vi "BrakeDelay (3).vi"(11 "Mtr Power":dbl) -> ()   [LabVIEW 2016]
uses:
  <vilib>/Rock Robotics/WPI/ThirdParty/CanMotor/TalonSRX/WPI_CANTalonSRX_BrakeOverride.ctl
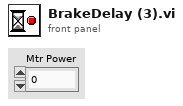
[diagram p1: front panel]
types:
  T1 = typedef "WPI_MotorControlDeviceRef.ctl" = cluster{"DeviceStatus":errorcluster, "Type":T2, "PWM":cluster{"PWM Channel":T3, "DeadBand":T4}, "CAN":cluster{"Device Number":u8, "SetOutput VI Ref":variant, "GetOutput VI Ref":variant, "Enable VI Ref":variant, "Disable VI Ref":variant, "Data":variant}, "Invert":bool}
  T2 = typedef "WPI_MotorControlType.ctl" = enum16{"PWM", "CAN"}
  T3 = typedef "FPGA_DIOPWMChannel.ctl" = enum8{"PWM 0", "PWM 1", "PWM 2", "PWM 3", "PWM 4", "PWM 5", "PWM 6", "PWM 7", "PWM 8", "PWM 9", "PWM MXP 0", "PWM MXP 1", "PWM MXP 2", "PWM MXP 3", "PWM MXP 4", "PWM MXP 5", "PWM MXP 6", "PWM MXP 7", "PWM MXP 8", "PWM MXP 9", "Invalid"}
  T4 = typedef "WPI_PWMDeadband.ctl" = cluster{"Name":string, "maxPositivePwm":i32, "minPositivePwm":i32, "centerPwm":i32, "maxNegativePwm":i32, "minNegativePwm":i32, "angularRange":u16}
  T5 = typedef "WPI_CANTalonSRX_BrakeOverride.ctl" = enum8{"No Override", "Override to Coast", "Override to Brake"}
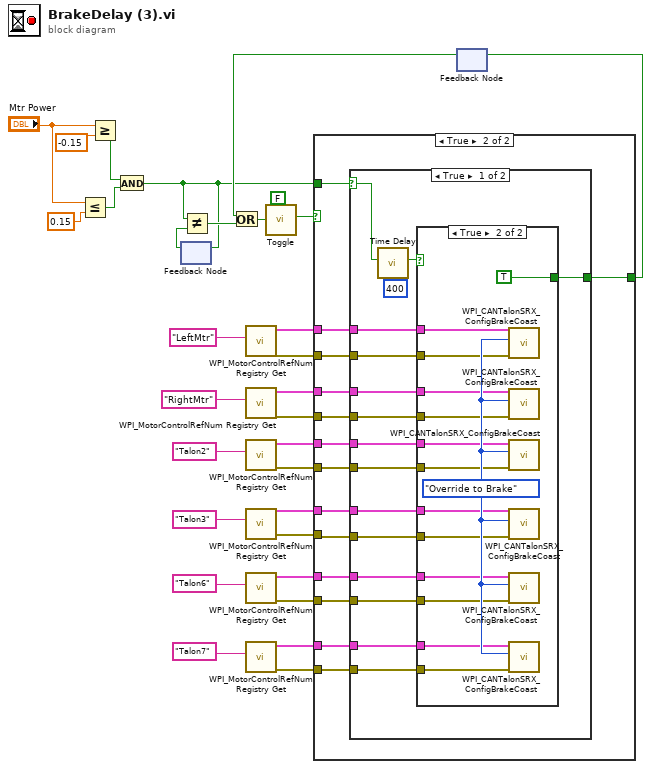
[diagram p0: block diagram]
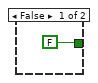
[diagram p2: hidden frame]
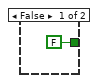
[diagram p3: hidden frame]
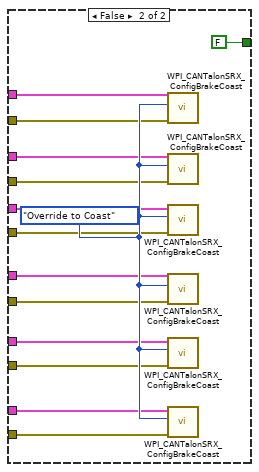
[diagram p4: hidden frame]
diagram:
  n1 = Less Or Equal?(x="Mtr Power", y=0.15) -> (x <= y?=w10:bool)
  n2 = Greater Or Equal?(x="Mtr Power", y=-0.15) -> (x >= y?=w9:bool)
  n3 = And(x=w9, y=w10) -> (x .and. y?=w2:bool)
  n4 = feedback #1() -> (w8:bool)  [unwired: 1 in]
  n5 = feedback-in #1(w2) -> ()
  n6 = Not Equal?(x=w2, y=w8) -> (x != y?=w7:bool)
  n7 = call <vilib>:"WPI_MotorControlRefNum Registry Get.vi"("refnum name"="LeftMtr") -> ("error out"=w30:errorcluster, "MotorControlDevRef"=w31:T1)  [unwired: 9 in]
  n8 = call <vilib>:"WPI_MotorControlRefNum Registry Get.vi"("refnum name"="RightMtr") -> ("error out"=w28:errorcluster, "MotorControlDevRef"=w29:T1)  [unwired: 9 in]
  n9 = call <vilib>:"WPI_MotorControlRefNum Registry Get.vi"("refnum name"="Talon2") -> ("error out"=w26:errorcluster, "MotorControlDevRef"=w27:T1)  [unwired: 9 in]
  n10 = call <vilib>:"WPI_MotorControlRefNum Registry Get.vi"("refnum name"="Talon3") -> ("error out"=w21:errorcluster, "MotorControlDevRef"=w20:T1)  [unwired: 9 in]
  n11 = call <vilib>:"WPI_MotorControlRefNum Registry Get.vi"("refnum name"="Talon6") -> ("error out"=w24:errorcluster, "MotorControlDevRef"=w25:T1)  [unwired: 9 in]
  n12 = call <vilib>:"WPI_MotorControlRefNum Registry Get.vi"("refnum name"="Talon7") -> ("error out"=w22:errorcluster, "MotorControlDevRef"=w23:T1)  [unwired: 9 in]
  n13 = feedback #2() -> (w3:bool)  [unwired: 1 in]
  n14 = Or(x=w3, y=w7) -> (x .or. y?=w6:bool)
  n15 = call "Toggle.vi"("Control"=FALSE, "Input"=w6) -> ("Output"=w5:bool)  [unwired: 9 in]
  n16 = case shown="True" w5 {
    tunnel: w20 -> [_ w41]
    tunnel: w21 -> [_ w42]
    tunnel: w22 -> [_ w46]
    tunnel: w23 -> [_ w45]
    tunnel: w24 -> [_ w44]
    tunnel: w25 -> [_ w43]
    tunnel: w26 -> [_ w40]
    tunnel: w27 -> [_ w39]
    tunnel: w28 -> [_ w38]
    tunnel: w29 -> [_ w37]
    tunnel: w30 -> [_ w36]
    tunnel: w31 -> [_ w35]
    tunnel: [FALSE w34] -> w4
    tunnel: w2 -> [_ w33]
    frame False {
    }
    frame True {
      n17 = case shown="True" w33 {
        selector: w33 -> [w50 _]
        tunnel: w46 -> [w62 w90]
        tunnel: w45 -> [w61 w89]
        tunnel: w44 -> [w60 w88]
        tunnel: w43 -> [w59 w87]
        tunnel: w42 -> [w58 w86]
        tunnel: w41 -> [w57 w85]
        tunnel: w40 -> [w56 w84]
        tunnel: w39 -> [w55 w83]
        tunnel: w38 -> [w54 w82]
        tunnel: w37 -> [w53 w81]
        tunnel: w36 -> [w52 w80]
        tunnel: w35 -> [w51 w79]
        tunnel: [w47 FALSE] -> w34
        frame True {
          n18 = call "Time Delay.vi"("Time Delay"=u32 400, "Boolean in"=w50) -> ("Boolean out"=w49:bool)  [unwired: 9 in]
          n19 = case shown="True" w49 {
            tunnel: w62 -> [_ w76]
            tunnel: w61 -> [_ w75]
            tunnel: w60 -> [_ w74]
            tunnel: w59 -> [_ w73]
            tunnel: w58 -> [_ w72]
            tunnel: w57 -> [_ w71]
            tunnel: w56 -> [_ w70]
            tunnel: w55 -> [_ w69]
            tunnel: w54 -> [_ w68]
            tunnel: w53 -> [_ w67]
            tunnel: w52 -> [_ w66]
            tunnel: w51 -> [_ w65]
            tunnel: [FALSE TRUE] -> w47
            frame False {
            }
            frame True {
              w77 = WPI_CANTalonSRX_BrakeOverride."Override to Brake" ("Brake / Coast Mode")
              n20 = call <vilib>:"WPI_CANTalonSRX_ConfigBrakeCoast.vi"("error in (no error)"=w66, "Brake / Coast Mode"=w77, "CAN Talon SRX Ref"=w65) -> ()  [unwired: 7 in, 2 out]
              n21 = call <vilib>:"WPI_CANTalonSRX_ConfigBrakeCoast.vi"("error in (no error)"=w68, "Brake / Coast Mode"=w77, "CAN Talon SRX Ref"=w67) -> ()  [unwired: 7 in, 2 out]
              n22 = call <vilib>:"WPI_CANTalonSRX_ConfigBrakeCoast.vi"("error in (no error)"=w70, "Brake / Coast Mode"=w77, "CAN Talon SRX Ref"=w69) -> ()  [unwired: 7 in, 2 out]
              n23 = call <vilib>:"WPI_CANTalonSRX_ConfigBrakeCoast.vi"("error in (no error)"=w72, "Brake / Coast Mode"=w77, "CAN Talon SRX Ref"=w71) -> ()  [unwired: 7 in, 2 out]
              n24 = call <vilib>:"WPI_CANTalonSRX_ConfigBrakeCoast.vi"("error in (no error)"=w74, "Brake / Coast Mode"=w77, "CAN Talon SRX Ref"=w73) -> ()  [unwired: 7 in, 2 out]
              n25 = call <vilib>:"WPI_CANTalonSRX_ConfigBrakeCoast.vi"("error in (no error)"=w76, "Brake / Coast Mode"=w77, "CAN Talon SRX Ref"=w75) -> ()  [unwired: 7 in, 2 out]
            }
          }
        }
        frame False {
          w91 = WPI_CANTalonSRX_BrakeOverride."Override to Coast" ("Brake / Coast Mode")
          n26 = call <vilib>:"WPI_CANTalonSRX_ConfigBrakeCoast.vi"("error in (no error)"=w80, "Brake / Coast Mode"=w91, "CAN Talon SRX Ref"=w79) -> ()  [unwired: 7 in, 2 out]
          n27 = call <vilib>:"WPI_CANTalonSRX_ConfigBrakeCoast.vi"("error in (no error)"=w82, "Brake / Coast Mode"=w91, "CAN Talon SRX Ref"=w81) -> ()  [unwired: 7 in, 2 out]
          n28 = call <vilib>:"WPI_CANTalonSRX_ConfigBrakeCoast.vi"("error in (no error)"=w84, "Brake / Coast Mode"=w91, "CAN Talon SRX Ref"=w83) -> ()  [unwired: 7 in, 2 out]
          n29 = call <vilib>:"WPI_CANTalonSRX_ConfigBrakeCoast.vi"("error in (no error)"=w86, "Brake / Coast Mode"=w91, "CAN Talon SRX Ref"=w85) -> ()  [unwired: 7 in, 2 out]
          n30 = call <vilib>:"WPI_CANTalonSRX_ConfigBrakeCoast.vi"("error in (no error)"=w88, "Brake / Coast Mode"=w91, "CAN Talon SRX Ref"=w87) -> ()  [unwired: 7 in, 2 out]
          n31 = call <vilib>:"WPI_CANTalonSRX_ConfigBrakeCoast.vi"("error in (no error)"=w90, "Brake / Coast Mode"=w91, "CAN Talon SRX Ref"=w89) -> ()  [unwired: 7 in, 2 out]
        }
      }
    }
  }
  n32 = feedback-in #2(w4) -> ()
